vi "Get Queue Ref.vi"(8 "error in (no error)":errorcluster, 11 "Stack in":refnum<class "Stack.lvclass">) -> (0 "error out":errorcluster, 2 "queue out":refnum<queue>, 3 "Stack out":refnum<class "Stack.lvclass">)   [LabVIEW 2016, in "Stack.lvlib" / "Stack.lvclass"]
doc: "This VI returns a queue reference. If not already exisiting the queue will be created."
uses:
  Stack.lvclass
  Stack.lvclass/Stack.ctl
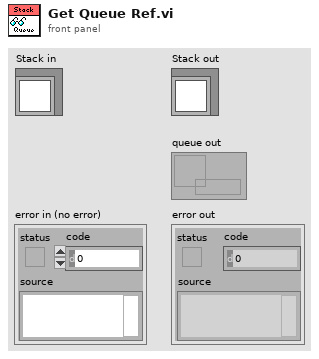
[diagram p1: front panel]
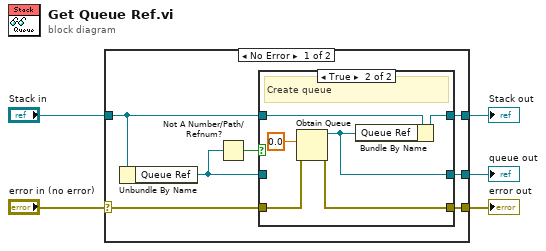
[diagram p0: block diagram]
diagram:
  n1 = case shown="No Error" "error in (no error)" {
    selector: "error in (no error)" -> [w7 w23]
    tunnel: [w6 w23] -> w4
    tunnel: [w10 w22] -> w2
    tunnel: "Stack in" -> [w11 w22]
    tunnel: [w9 _] -> w1
    frame No Error {
      n2 = Unbundle By Name(w11) -> ("Queue Ref"=w8:refnum<queue>)
      n3 = Not A Number/Path/Refnum?(number/path/refnum=w8) -> (NaN/Path/Refnum?=w12:bool)
      n4 = case shown="True" w12 {
        tunnel: w11 -> [w15 w20]
        tunnel: [w15 w19] -> w10
        tunnel: [w14 w18] -> w9
        tunnel: w8 -> [w14 _]
        tunnel: w7 -> [w13 w17]
        tunnel: [w13 w16] -> w6
        frame False {
          # "Return exisiting queue"
        }
        frame True {
          # "Create queue"
          n5 = Obtain Queue(element data type=0.0, error in (no error)=w17) -> (queue out=w18:refnum<queue>, error out=w16:errorcluster)  [unwired: 3 in, 1 out]
          n6 = Bundle By Name(cluster=w20, "Queue Ref"=w18) -> (w19:refnum<class "Stack.lvclass">)
        }
      }
    }
    frame Error {
    }
  }
  "error out" <- w4
  "Stack out" <- w2
  "queue out" <- w1
